vi "Temperature controller.vi"() -> ()   [LabVIEW 2010]
panel:
  in  "Set point":sgl format="%.3f"
  in  "stop":bool
  out "Current temperature":sgl format="%.3f"
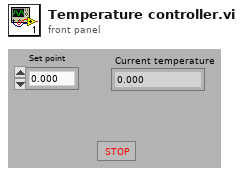
[diagram p1: front panel]
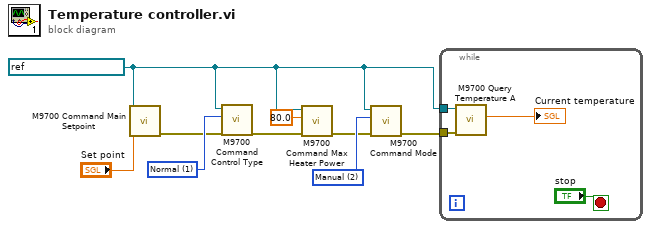
[diagram p0: block diagram]
diagram:
  w4 = u16 2 items=["None", "Stop", "Manual", "Program", "Autotune", "Fixed Output"] ("uiMode")
  w8 = u16 1 items=["None", "Normal", "Zone"] ("uiType")
  w1 = refnum<visa-resource-name> "GPIB0::15::INSTR" ("VISA Resource Name")
  n1 = call <instrlib>:"M9700 Command Main Setpoint.vi"("flMainSet"="Set point", "VISA Resource Name"=w1) -> ("error out"=w7:errorcluster)  [unwired: 8 in, 1 out]
  n2 = call <instrlib>:"M9700 Command Control Type.vi"("error in (no error)"=w7, "uiType"=w8, "VISA Resource Name"=w1) -> ("error out"=w5:errorcluster)  [unwired: 7 in, 1 out]
  n3 = call <instrlib>:"M9700 Command Max Heater Power.vi"("error in (no error)"=w5, "flMax_Heat"=sgl 80.0, "VISA Resource Name"=w1) -> ("error out"=w3:errorcluster)  [unwired: 7 in, 1 out]
  n4 = call <instrlib>:"M9700 Command Mode.vi"("error in (no error)"=w3, "uiMode"=w4, "VISA Resource Name"=w1) -> ("error out"=w2:errorcluster)  [unwired: 7 in, 1 out]
  n5 = while {
    tunnel: w1 -> [w13]
    tunnel: w2 -> [w10]
    stop <- "stop" stop-if-true
    n6 = call <instrlib>:"M9700 Query Temperature A.vi"("error in (no error)"=w10, "VISA Resource Name"=w13) -> ("flTempA"=→"Current temperature":sgl)  [unwired: 7 in, 2 out]
  }
